vi "Actor Core.vi"(8 "error in":errorcluster, 11 "Assert in":refnum<class "Assert.lvclass">) -> (0 "error out":errorcluster, 3 "Actor out":refnum<class "Actor.lvclass">)   [LabVIEW 2019, in "Assert.lvlib" / "Assert.lvclass"]
doc: "(<B>Filename</B>: Actor Framework.lvlib:Actor.lvclass:Actor Core.vi)\n\nReceives messages to the actor, reacts to them, and initiates any error handling that may shut the actor down.\n\nDescendant classes may override this VI to append parallel tasks for the actor to complete while it handles messages. Overrides use the Call Parent Method node."
uses:
  Assert.lvclass
  C:/Program Files (x86)/National Instruments/LabVIEW 2019/vi.lib/ActorFramework/Actor/Actor.lvclass
  <vilib>/ActorFramework/Actor/Actor.lvclass
  Assert.lvclass/Assert.ctl
  <vilib>/ActorFramework/Actor/Actor.lvclass/Actor.ctl
  <vilib>/ActorFramework/Message Enqueuer/Message Enqueuer.lvclass/Message Enqueuer.ctl
  Assert Event.lvclass
  C:/Program Files (x86)/National Instruments/LabVIEW 2019/vi.lib/NI/Event Source Actor/Event Source/Event/Event.lvclass
  <vilib>/NI/Event Source Actor/Event Source/Event/Event.lvclass/Event.ctl
  <vilib>/NI/Event Source Actor/Event Source/Event Source Messages/Generate Event Msg/Generate Event Msg.lvclass/Generate Event Msg.ctl
  <vilib>/ActorFramework/Message Enqueuer/Init from Existing Queue.vi
  <vilib>/ActorFramework/Message Enqueuer/Enqueue.vi
  <vilib>/NI/Event Source Actor/Event Source/Event Source Messages/Generate Event Msg/Generate Event Msg.lvclass
  C:/Program Files (x86)/National Instruments/LabVIEW 2019/vi.lib/ActorFramework/Message/Message.lvclass
  Unit Test Engine Global.vi
  <vilib>/ActorFramework/Message Priority Queue/Priority Enqueue.vi
  <vilib>/NI/Event Source Actor/Event Source/Event Source/Event Source.lvclass
  <vilib>/ActorFramework/Message Enqueuer/Message Enqueuer.lvclass
  Assert.lvlib
  <vilib>/NI/Event Source Actor/Event Source/Event/Event.lvclass
panel:
  out "StartTime":u32
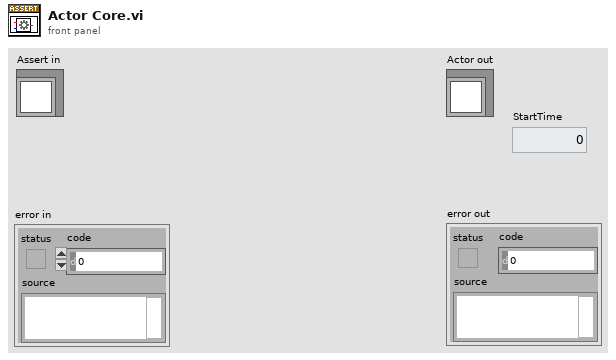
[diagram p1: front panel]
types:
  T1 = cluster{"Socket":i32, "Result":string, "Value":string, "Limit":cluster{"High":string, "Low":string}, "Type":string, "StepName":string, "Normal":string, "Unit":string}
  T2 = cluster{"Socket":i32, "StepName":string, "Sequence":string}
  T3 = enum32{"Invalid", "Standard", "Closed", "Hidden", "Minimized", "Maximized"}
  T4 = enum32{"invalid app kind", "Development System", "Run Time System", "Student Edition", "Embedded LabVIEW", "Evaluation", "Custom"}
  T5 = cluster{"Core":cluster{"Current VI Reference":refnum<vi>, "Close Panel on Exit?":bool}, "Your Boolean data":bool, "Your string data":string}
  T6 = cluster{"Current VI Reference":refnum<vi>, "Close Panel on Exit?":bool}
  T7 = cluster{"Socket":i32, "StepName":string, "Sequence":string}[]
  T8 = cluster{"Socket":i32, "Result":string, "Value":string, "Limit":cluster{"High":string, "Low":string}, "Type":string, "StepName":string, "Normal":string, "Unit":string}[]
  T9 = cluster{cluster{"Socket":i32, "Result":string, "Value":string, "Limit":cluster{"High":string, "Low":string}, "Type":string, "StepName":string, "Normal":string, "Unit":string}[], dbl}
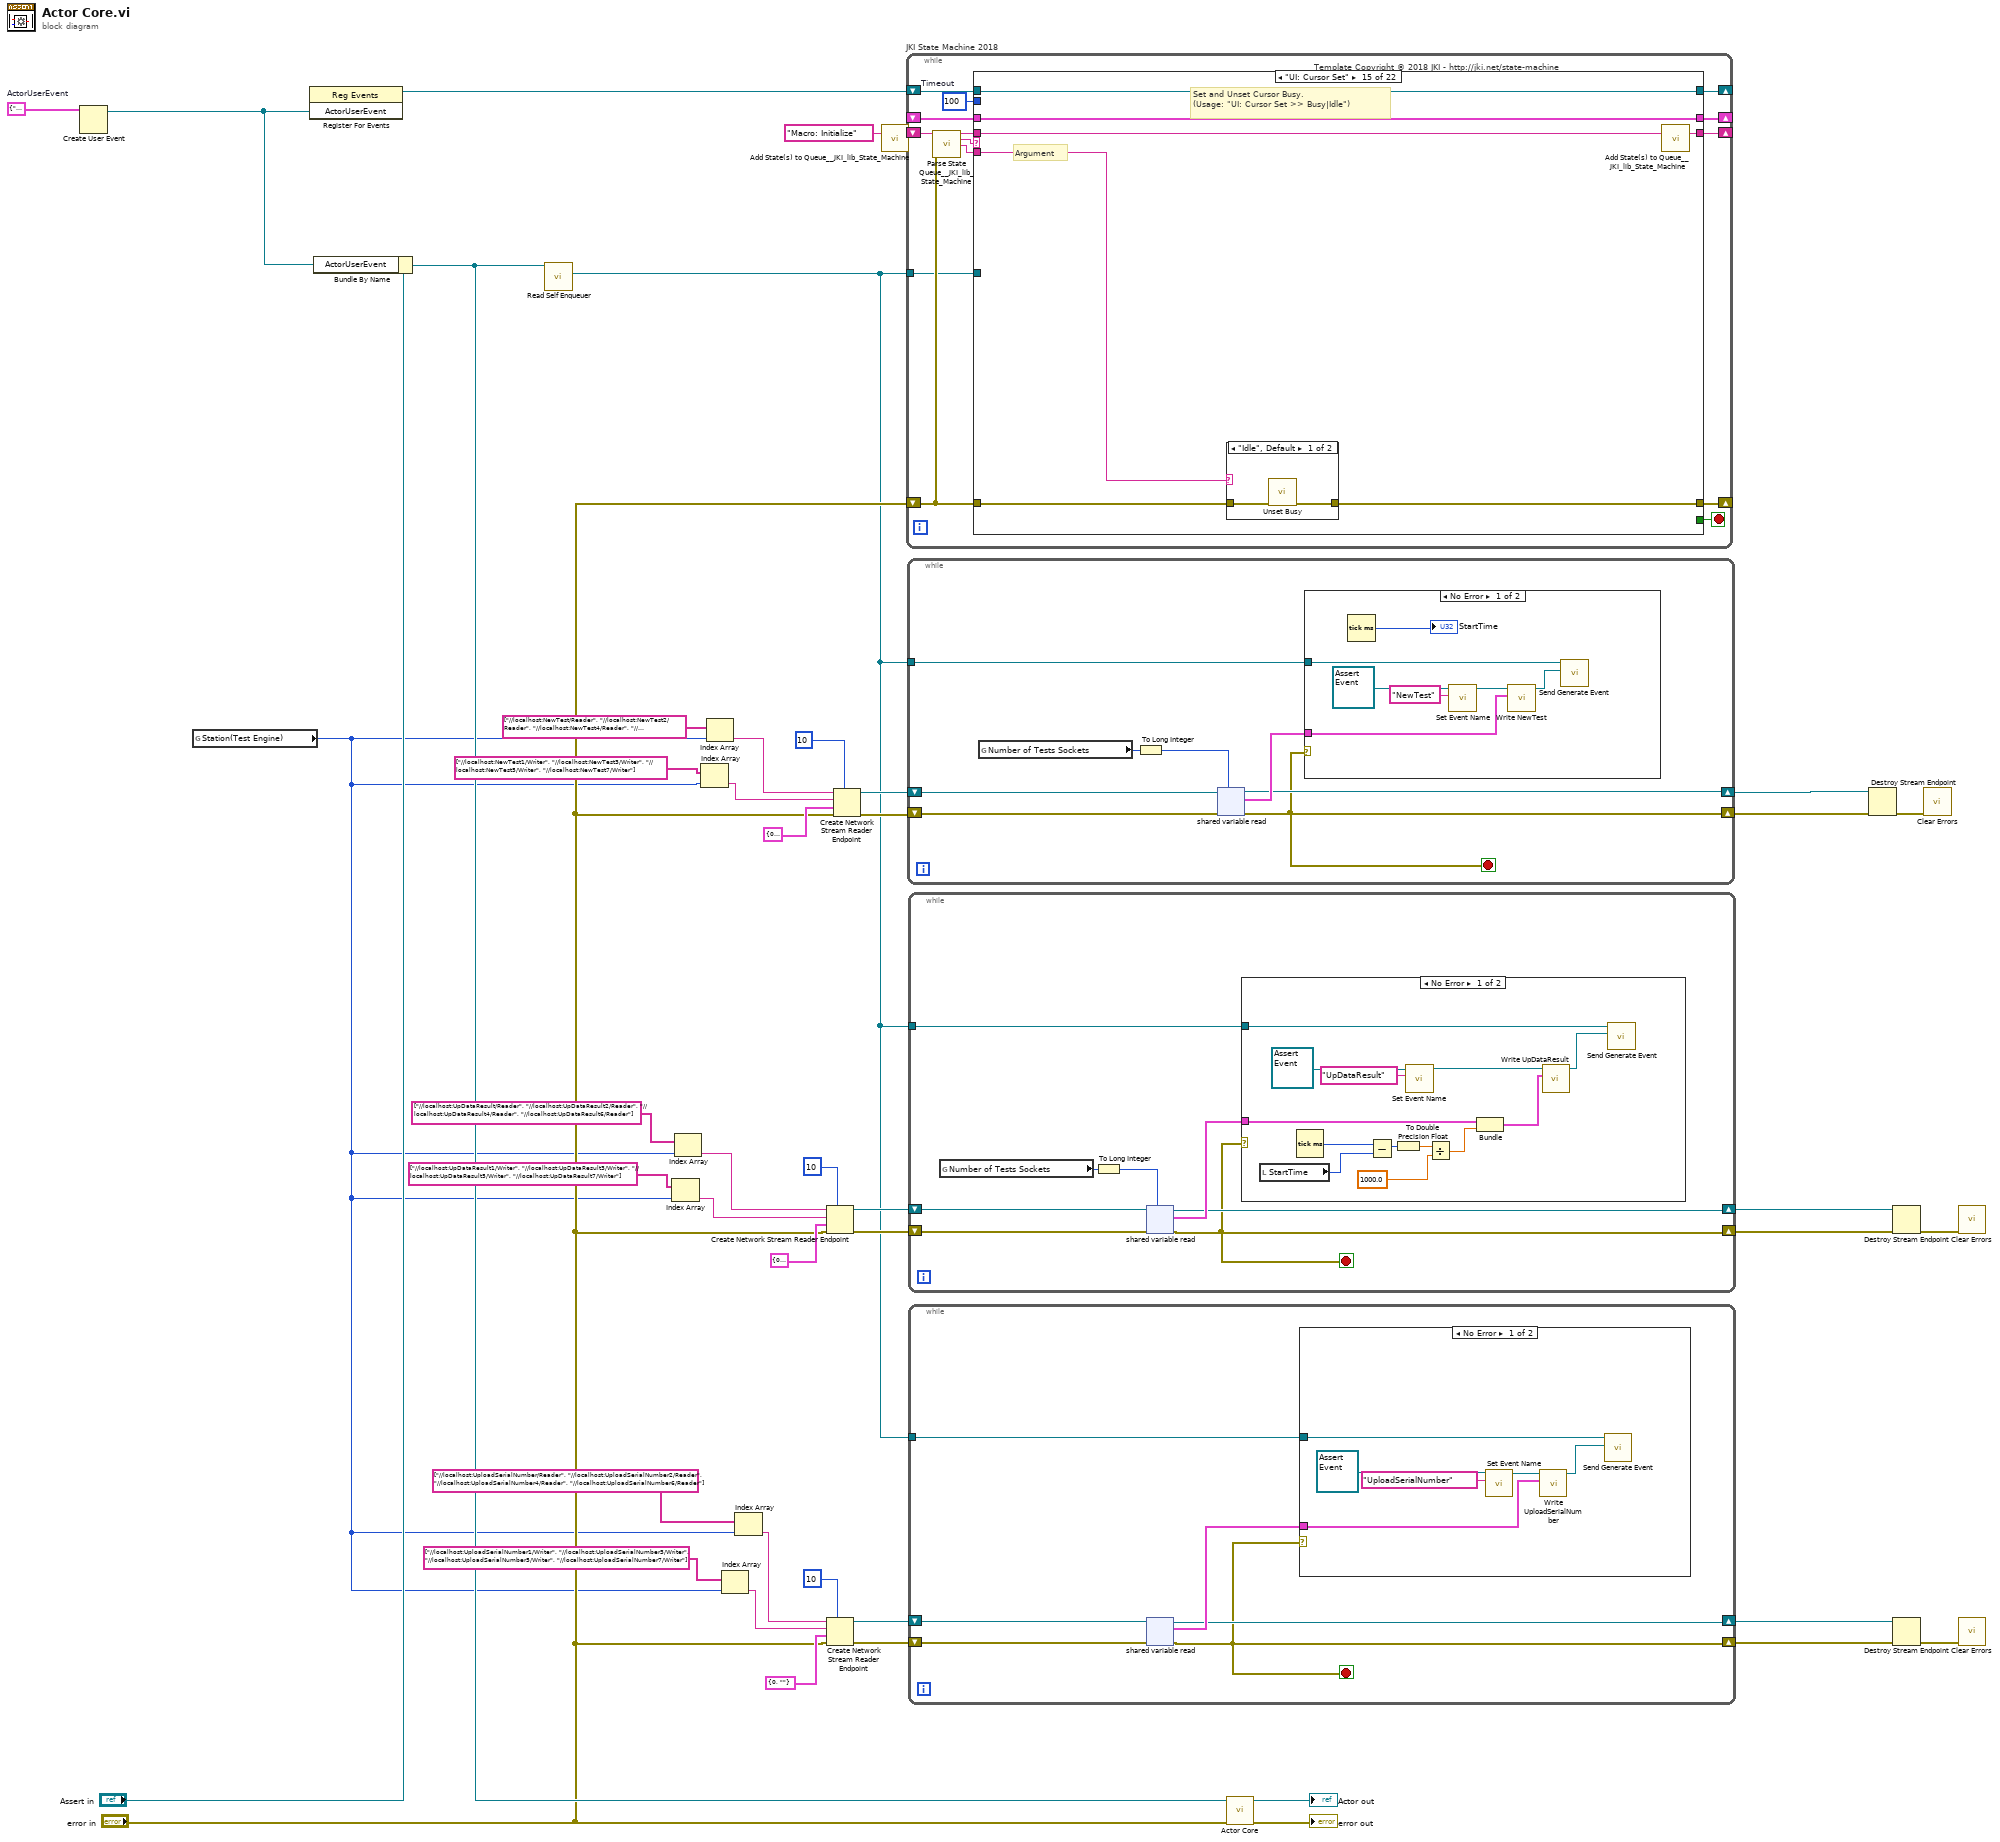
[diagram p0: block diagram]
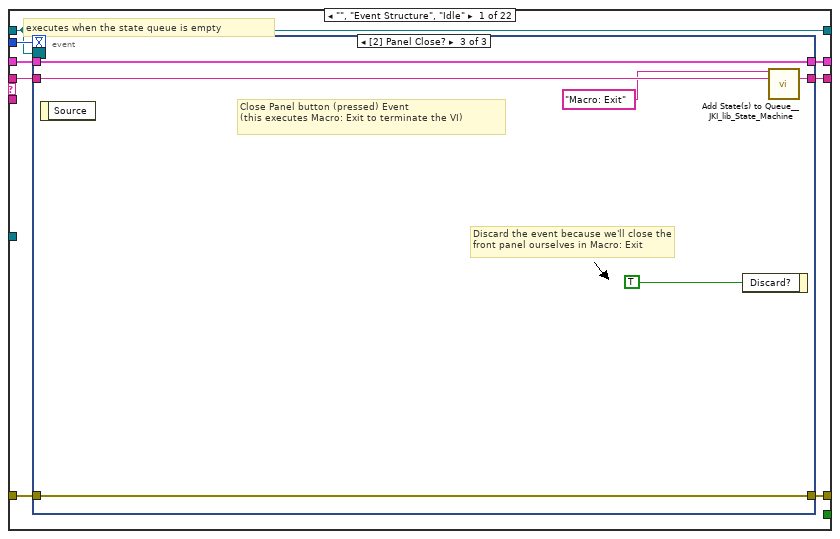
[diagram p5: hidden frame]
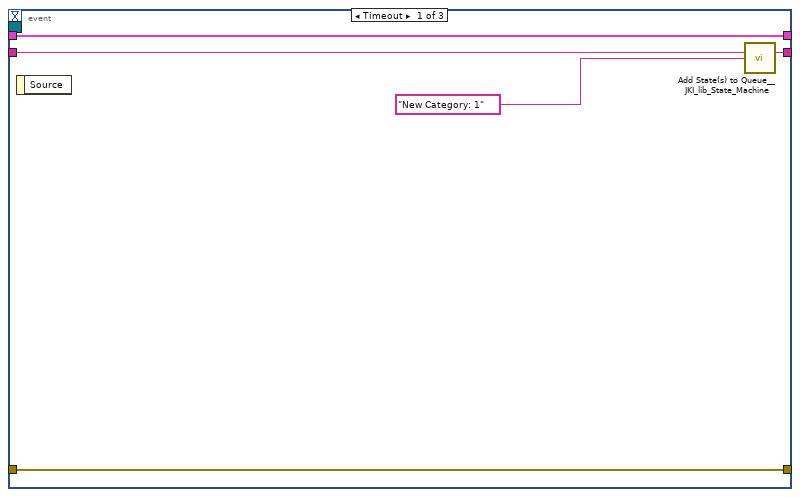
[diagram p6: hidden frame]
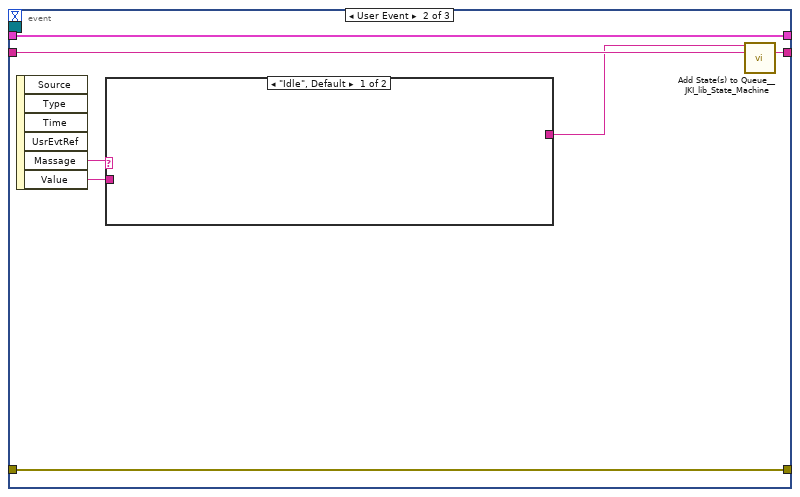
[diagram p7: hidden frame]
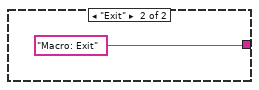
[diagram p8: hidden frame]
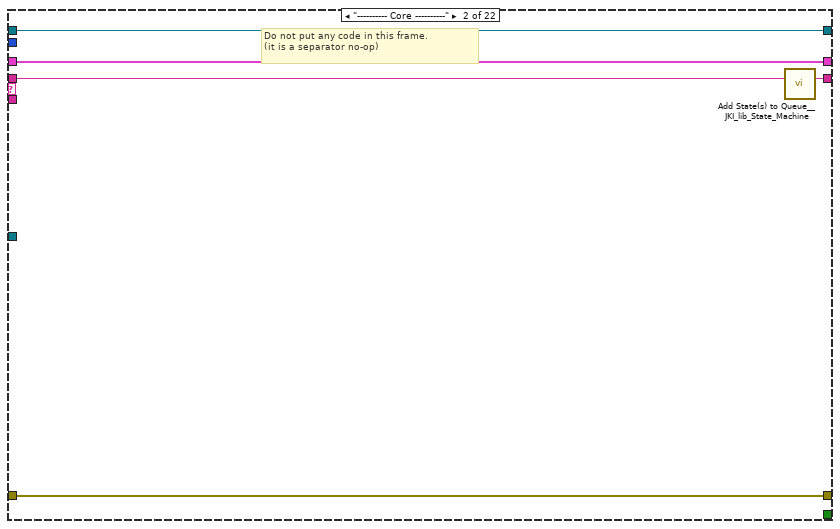
[diagram p9: hidden frame]
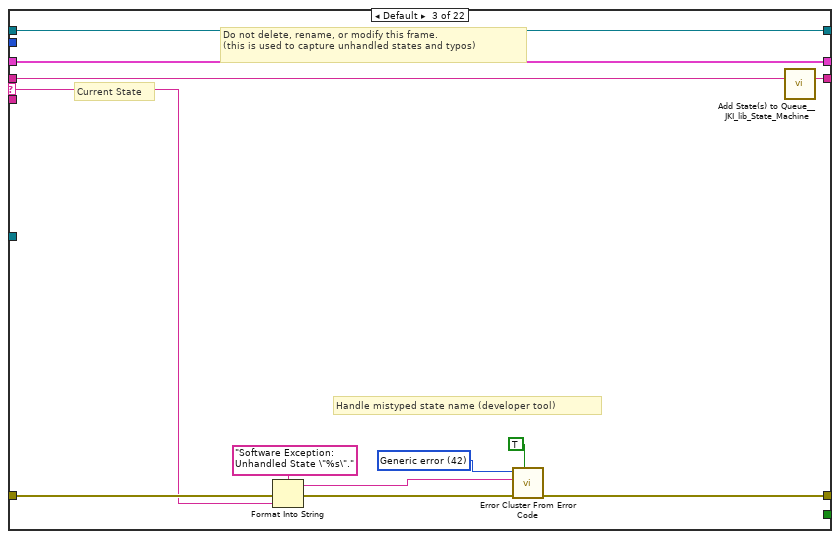
[diagram p10: hidden frame]
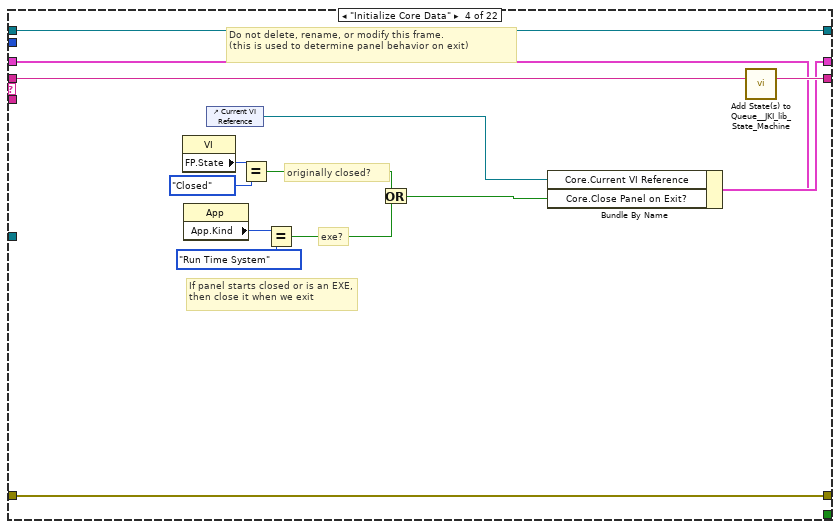
[diagram p11: hidden frame]
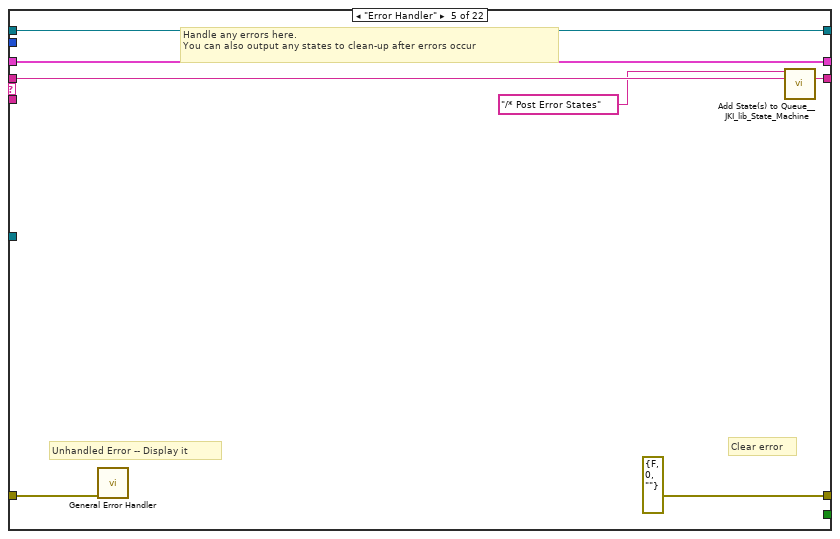
[diagram p12: hidden frame]
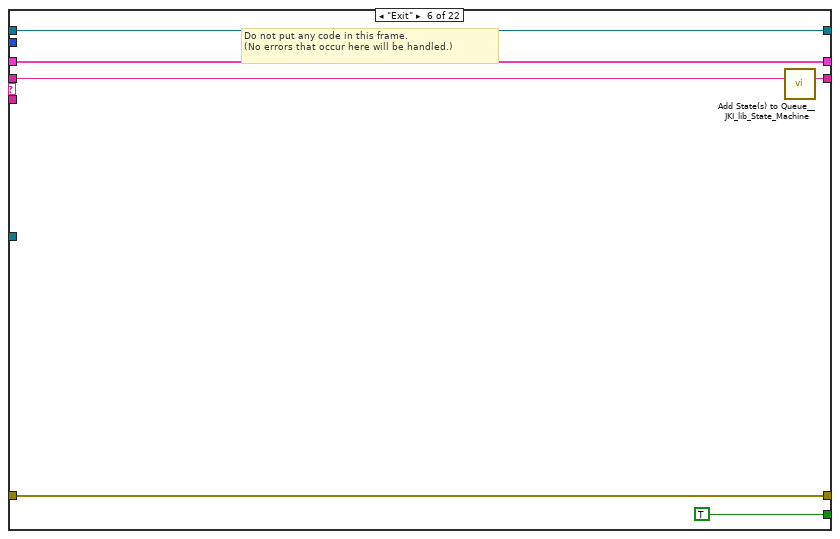
[diagram p13: hidden frame]
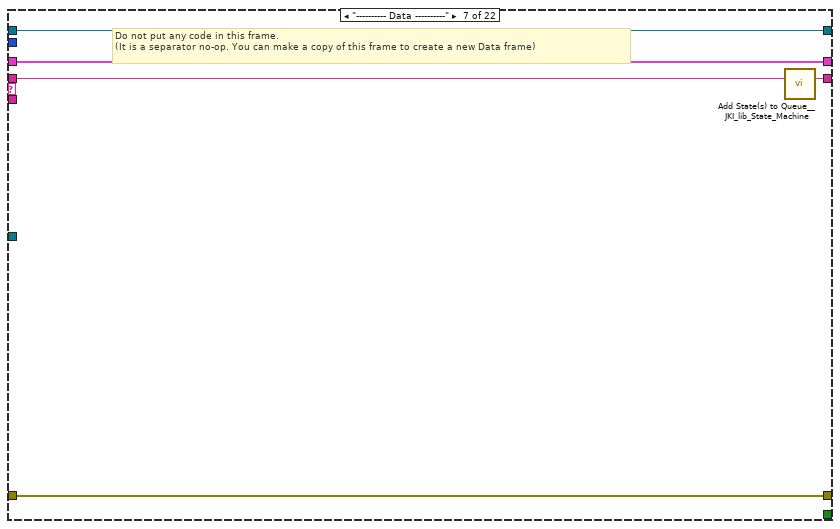
[diagram p14: hidden frame]
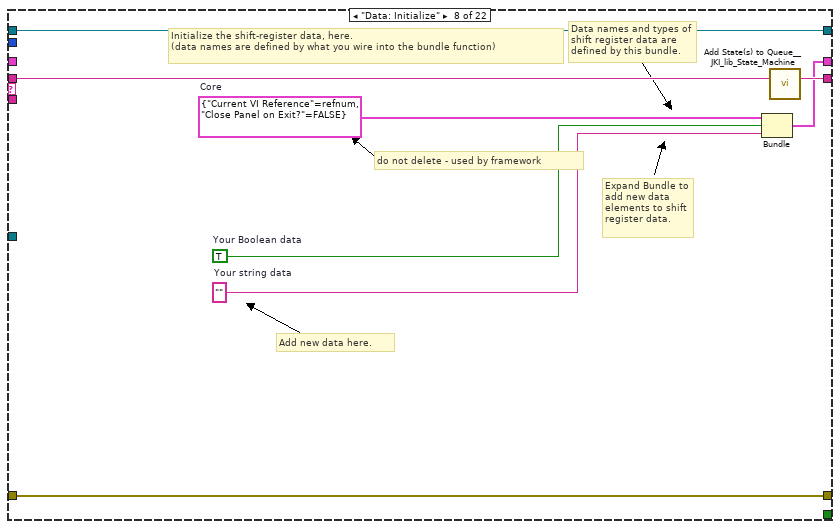
[diagram p15: hidden frame]
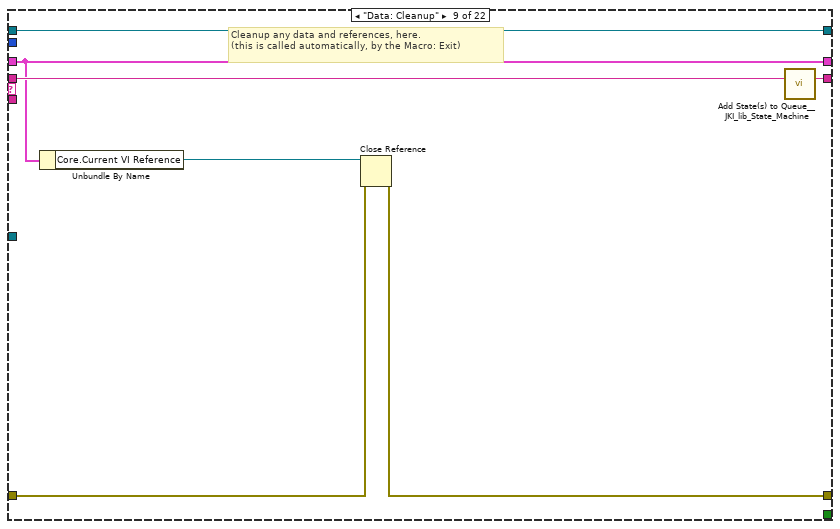
[diagram p16: hidden frame]
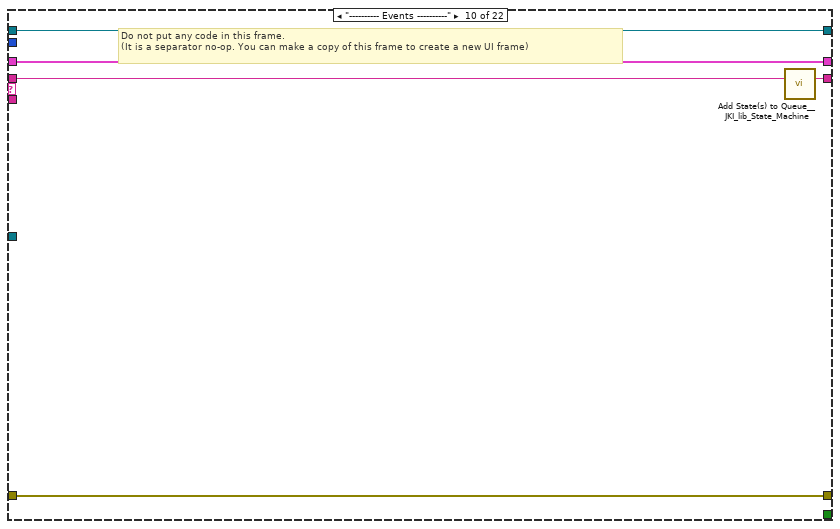
[diagram p17: hidden frame]
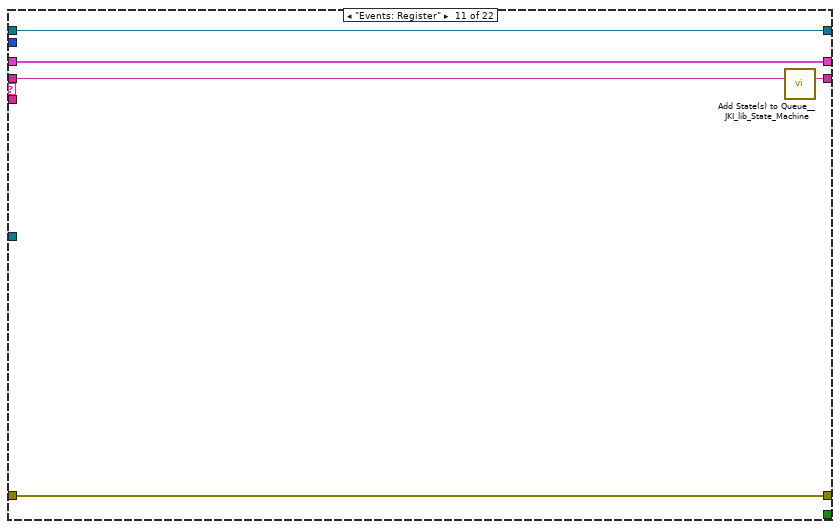
[diagram p18: hidden frame]
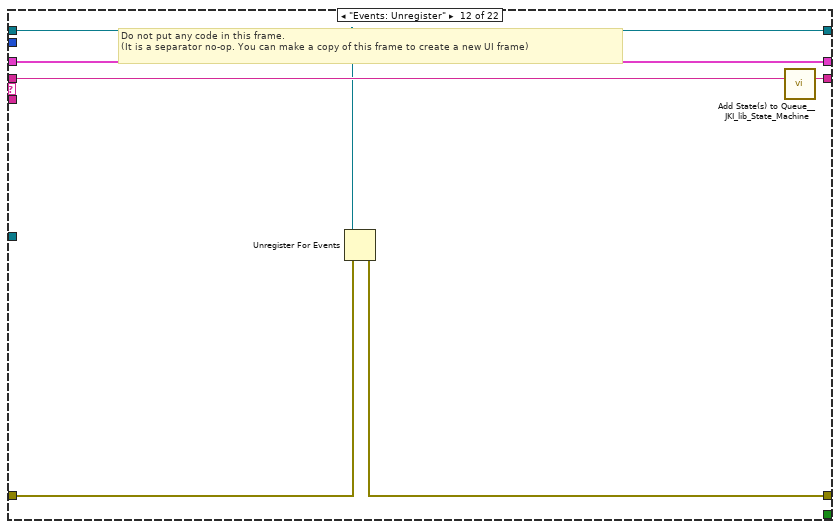
[diagram p19: hidden frame]
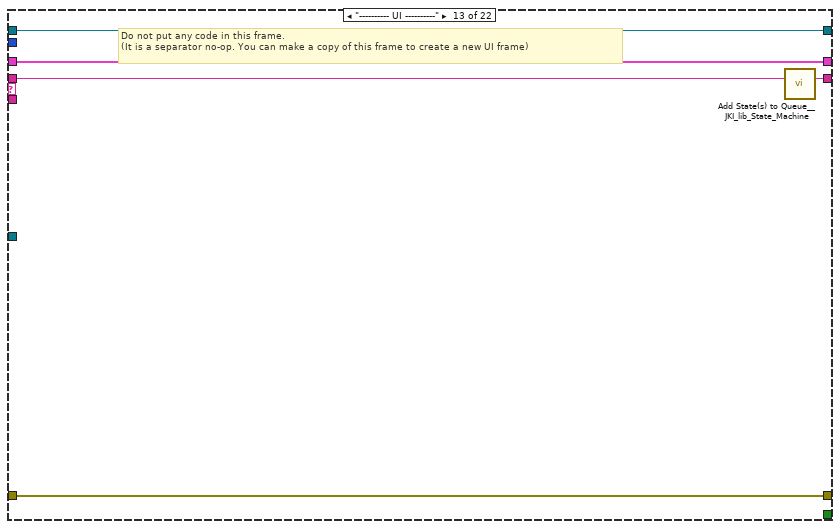
[diagram p20: hidden frame]
diagram:
  w41 = cluster{"Massage":string, "Value":string} {"Massage"="", "Value"=""}  # ActorUserEvent
  n1 = Create User Event(user event datatype=w41) -> (user event=w38:refnum<user-event>)  [unwired: 1 in, 1 out]
  n2 = global read "Unit Test Engine Global.vi" "Station(Test Engine)"() -> (w3:i32)
  n3 = register-events(w38) -> (reference out=w40:refnum<event-registration>)  [unwired: 2 in, 1 out]
  n4 = Bundle By Name(cluster="Assert in", "ActorUserEvent"=w38) -> (w16:refnum<class "Assert.lvclass">)
  n5 = call <vilib>:"Read Self Enqueuer.vi"("Actor"=w16) -> ("Self Enqueuer"=w1:refnum<class "Message Enqueuer.lvclass">)  [unwired: 10 in]
  n6 = Index Array(array=string[] ["//localhost:UpDataResult1/Writer", "//localhost:UpDataResult3/Writer", "//localhost:UpDataResult5/Writer", "//localhost:UpDataResult7/Writer"], index=w3) -> (element=w7:string)
  n7 = Index Array(array=string[] ["//localhost:UpDataResult/Reader", "//localhost:UpDataResult2/Reader", "//localhost:UpDataResult4/Reader", "//localhost:UpDataResult6/Reader"], index=w3) -> (element=w11:string)
  n8 = Index Array(array=string[] ["//localhost:NewTest1/Writer", "//localhost:NewTest3/Writer", "//localhost:NewTest5/Writer", "//localhost:NewTest7/Writer"], index=w3) -> (element=w2:string)
  n9 = Index Array(array=string[] ["//localhost:NewTest/Reader", "//localhost:NewTest2/Reader", "//localhost:NewTest4/Reader", "//localhost:NewTest6/Reader"], index=w3) -> (element=w13:string)
  n10 = Index Array(array=string[] ["//localhost:UploadSerialNumber1/Writer", "//localhost:UploadSerialNumber3/Writer", "//localhost:UploadSerialNumber5/Writer", "//localhost:UploadSerialNumber7/Writer"], index=w3) -> (element=w5:string)
  n11 = Index Array(array=string[] ["//localhost:UploadSerialNumber/Reader", "//localhost:UploadSerialNumber2/Reader", "//localhost:UploadSerialNumber4/Reader", "//localhost:UploadSerialNumber6/Reader"], index=w3) -> (element=w9:string)
  n12 = Create Network Stream Reader Endpoint(7:10 ("reader buffer size"), 8:"error in", 9:T1 {"Socket"=0, "Result"="", "Value"="", "Limit"={"High"="", "Low"=""}, "Type"="", "StepName"="", "Normal"="", "Unit"=""}, 10:w7, 11:w11) -> (0:w27:errorcluster, 3:w26:refnum<k21>)  [unwired: 2 in]
  n13 = Create Network Stream Reader Endpoint(7:10 ("reader buffer size"), 8:"error in", 9:cluster{"Socket":i32, "SerialNumber":string} {"Socket"=0, "SerialNumber"=""}, 10:w5, 11:w9) -> (0:w21:errorcluster, 3:w22:refnum<k21>)  [unwired: 2 in]
  n14 = Create Network Stream Reader Endpoint(7:10 ("reader buffer size"), 8:"error in", 9:T2 {"Socket"=0, "StepName"="", "Sequence"=""}, 10:w2, 11:w13) -> (0:w33:errorcluster, 3:w32:refnum<k21>)  [unwired: 2 in]
  n15 = call <vilib>:"Add State(s) to Queue__JKI_lib_State_Machine.vi"("State(s) in (\"\")"="Macro: Initialize") -> ("States Out"=w43:string)  [unwired: 14 in]
  n16 = while "JKI State Machine 2018" {
    shift-right: [w52] -> _
    shift-left: _ -> [w51]
    shift-right: [w55] -> _
    shift-left: "error in" -> [w49]
    shift-right: [w54] -> _
    shift-left: w43 -> [w56]
    shift-right: [w48] -> _
    shift-left: w40 -> [w47]
    tunnel: w1 -> [w46]
    stop <- w53 stop-if-true
    w50 = 100  # Timeout
    # "Template Copyright © 2018 JKI - http://jki.net/state-machine"
    n17 = call <vilib>:"Parse State Queue__JKI_lib_State_Machine.vi"("State Queue"=w56, "Error In (no error)"=w49) -> ("Remaining States"=w58:string, "Current State"=w59:string, "Arguments"=w57:string)  [unwired: 11 in]
    n18 = case shown="\"UI: Cursor Set\"" w59 {
      selector: w59 -> [_ _ w93 _ _ _ _ _ _ _ _ _ _ _ _ _ _ _ _ _ _ _]
      tunnel: w58 -> [w67 w91 w97 w117 w124 w130 w135 w143 w150 w155 w160 w166 w171 w176 w183 w195 w265 w271 w282 w287 w292 w297]
      tunnel: w57 -> [_ _ _ _ _ _ _ _ _ _ _ _ _ _ w178 w189 _ _ _ _ _ _]
      tunnel: w51 -> [w65 w88 w95 w110 w121 w128 w132 _ w145 w152 w158 w164 w168 w174 w181 w191 w262 w268 w279 w284 w290 w294]
      tunnel: [w64 w89 w99 w114 errorcluster {"status"=FALSE, "code"=0, "source"=""} ("error out") w127 w133 w140 w146 w153 w157 w161 w169 w173 w179 w192 w263 w269 w280 w285 w288 w295] -> w55
      tunnel: w49 -> [w63 w89 w98 w114 w120 w127 w133 w140 w147 w153 w157 w162 w169 w173 w180 w193 w263 w269 w280 w285 w288 w295]
      tunnel: [w66 w90 w96 w116 w123 w129 w134 w142 w149 w154 w159 w165 w170 w175 w182 w194 w264 w270 w281 w286 w291 w296] -> w54
      tunnel: [_ _ _ _ _ TRUE _ _ _ _ _ _ _ _ _ _ _ _ _ _ _ _] -> w53
      tunnel: [w62 w88 w95 w115 w121 w128 w132 w141 w145 w152 w158 w164 w168 w174 w181 w191 w262 w268 w279 w284 w290 w294] -> w52
      tunnel: w50 -> [w61 _ _ _ _ _ _ _ _ _ _ _ _ _ _ _ _ _ _ _ _ _]
      tunnel: [w60 w87 w92 w104 w118 w125 w131 w136 w144 w151 w156 w163 w167 w172 w177 w188 w261 w266 w272 w283 w289 w293] -> w48
      tunnel: w47 -> [w60 w87 w92 w104 w118 w125 w131 w136 w144 w151 w156 w163 w167 w172 w177 w188 w261 w266 w272 w283 w289 w293]
      tunnel: w46 -> [_ _ _ _ _ _ _ _ _ _ _ _ _ _ _ _ _ _ _ _ _ _]
      frame "", "Event Structure", "Idle" {
        # "executes when the state queue is empty"
        n19 = event shown="[2] Panel Close?" {
          selector: w60 -> [_ _ _]
          dyn-events: _ -> [_ _ _]
          timeout: w61 -> [_ _ _]
          tunnel: w67 -> [w72 w79 w86]
          tunnel: [w71 w78 w85] -> w66
          tunnel: w65 -> [w69 w76 w83]
          tunnel: [w70 w77 w84] -> w64
          tunnel: w63 -> [w70 w77 w84]
          tunnel: [w69 w76 w83] -> w62
          event Timeout {
            n20 = event-data() -> ()  [unwired: 1 in, 1 out]
            n21 = call <vilib>:"Add State(s) to Queue__JKI_lib_State_Machine.vi"("State(s) in (\"\")"=w72, "State(s) at Back (\"\")"="New Category: 1" ("State(s) at Back (\"\")")) -> ("States Out"=w71:string)  [unwired: 13 in]
          }
          event User Event {
            n22 = event-data() -> ("Massage"=w75:string, "Value"=w73:string)  [unwired: 1 in, 4 out]
            n23 = case shown="\"Idle\", Default" w75 {
              tunnel: [_ "Macro: Exit"] -> w74
              tunnel: w73 -> [_ _]
              frame "Idle", Default {
              }
              frame "Exit" {
              }
            }
            n24 = call <vilib>:"Add State(s) to Queue__JKI_lib_State_Machine.vi"("State(s) in Front (\"\")"=w74, "State(s) in (\"\")"=w79) -> ("States Out"=w78:string)  [unwired: 13 in]
          }
          event Panel Close? {
            # "Discard the event because we'll close the front panel ourselves in Macro: Exit"
            # "Close Panel button (pressed) Event\n(this executes Macro: Exit to terminate the VI)"
            n25 = event-data() -> ()  [unwired: 1 in, 1 out]
            n26 = event-data("Discard?"=TRUE) -> ()  [unwired: 1 in, 1 out]
            n27 = call <vilib>:"Add State(s) to Queue__JKI_lib_State_Machine.vi"("State(s) in Front (\"\")"="Macro: Exit", "State(s) in (\"\")"=w86) -> ("States Out"=w85:string)  [unwired: 13 in]
          }
        }
      }
      frame "---------- Core ----------" {
        # "Do not put any code in this frame.\n(it is a separator no-op)"
        n28 = call <vilib>:"Add State(s) to Queue__JKI_lib_State_Machine.vi"("State(s) in (\"\")"=w91) -> ("States Out"=w90:string)  [unwired: 14 in]
      }
      frame Default {
        w102 = 42 items=["No error", "Argument error", "Memory is full", "Out of zone", "End of file", "File already open", "Generic file I/O error", "File not found", "File permission error", "Disk is full", "Duplicate path", "Too many files open", "System feature not enabled", "Resource file not found", "Cannot add resource", "Resource not found", "Image not found", "Image memory error", "Pen does not exist", "Config type invalid", "Config token not found", "Config parse error", "Config memory error", "Bad external code format", "Bad external code offset", "External code not present", "Null window", "Destroy window error", "Null menu", "Print aborted", "Bad print record", "Print driver error", "Windows error during printing", "Memory error during printing", "Print dialog error", "Generic print error", "Invalid device refnum", "Device not found", "Device parameter error", "Device unit error", "Cannot open device", "Device call aborted", "Generic error", "Cancelled by user", "Object ID too low", "Object ID too high", "Object not in heap", "Unknown heap", "Unknown object (invalid DefProc)", "Unknown object (DefProc not in table)", "Message out of range", "Invalid (null) method", "Unknown message", "Manager call not supported", "Bad address", "Network operation in progress", "Network operation timed out", "Connection is busy", "Network attribute not supported", "Network error", "Address in use", "System out of memory", "Connection aborted", "Connection refused", "Not connected", "Already connected", "Connection closed", "Initialization error (interapplication manager)", "Bad occurrence", "Wait on unbound occurrence handler", "Occurrence queue overflow", "Datalog type conflict", "Unused", "Unrecognized type (interapplication manager)", "Memory corrupt", "Failed to make temporary DLL", "Old CIN version", "Drag socket not found", "Failed to load drop-object", "Failed to register OLE object", "Failed to release OLE object", "Format specifier type mismatch", "Unknown format specifier", "Too few format specifiers", "Too many format specifiers", "Scan failed", "Newer CIN version", "Error converting to variant", "Runtime menu error", "Password tampered", "Variant attribute not found", "Incompatible variant data type", "Event data is not available", "Event Store is not present", "Occurrence is not found", "Event Queue is not created", "Event info is not available", "Refnum passed is NULL", "Error retrieving Class GUID", "Error retrieving CoClass GUID", "Error retrieving TypeLib GUID.", "Bad built application magic bytes.", "Specific driver is different from the specific driver associated with the Logical Name.", "There is no session opened to the class driver.", "Max Error", "MAX - Error with config objects", "MAX - Error loading configuration", "MAX - Group not supported"]
        # "Current State"
        # "Do not delete, rename, or modify this frame.\n(this is used to capture unhandled states and typos)"
        # "Handle mistyped state name (developer tool)"
        n29 = Format Into String(format string="Software Exception: Unhandled State \"%s\"." ("message"), error in=w98, w93) -> (resulting string=w101:string, error out=w100:errorcluster)  [unwired: 1 in]
        n30 = call <vilib>:"Error Cluster From Error Code.vi"("show call chain? (False)"=TRUE, "error in (no error)"=w100, "error message (\"\")"=w101, "error code (0)"=w102) -> ("error out"=w99:errorcluster)  [unwired: 5 in]
        n31 = call <vilib>:"Add State(s) to Queue__JKI_lib_State_Machine.vi"("State(s) in (\"\")"=w97) -> ("States Out"=w96:string)  [unwired: 14 in]
      }
      frame "Initialize Core Data" {
        # "Do not delete, rename, or modify this frame.\n(this is used to determine panel behavior on exit)"
        # "originally closed?"
        # "exe?"
        # "If panel starts closed or is an EXE, then close it when we exit"
        n32 = property class="VI"() -> ("FP.State"=w107:T3)  [unwired: 2 in, 2 out]
        n33 = property class="App"() -> ("App.Kind"=w113:T4)  [unwired: 2 in, 2 out]
        n34 = control-ref of="Current VI Reference"() -> (w108:refnum<vi>)
        n35 = Equal?(x=w107, y=T3."Closed" ("Front Panel Window:State")) -> (x = y?=w105:bool)
        n36 = Equal?(x=w113, y=T4."Run Time System" ("Application:Kind")) -> (x = y?=w111:bool)
        n37 = Or(x=w105, y=w111) -> (x .or. y?=w109:bool)
        n38 = Bundle By Name(cluster=w110, "Core.Current VI Reference"=w108, "Core.Close Panel on Exit?"=w109) -> (w115:T5)
        n39 = call <vilib>:"Add State(s) to Queue__JKI_lib_State_Machine.vi"("State(s) in (\"\")"=w117) -> ("States Out"=w116:string)  [unwired: 14 in]
      }
      frame "Error Handler" {
        # "Unhandled Error -- Display it"
        # "Handle any errors here.\nYou can also output any states to clean-up after errors occur"
        # "Clear error"
        n40 = call <vilib>:"General Error Handler.vi"("error in (no error)"=w120) -> ()  [unwired: 10 in, 5 out]
        n41 = call <vilib>:"Add State(s) to Queue__JKI_lib_State_Machine.vi"("State(s) in Front (\"\")"="/* Post Error States", "State(s) in (\"\")"=w124) -> ("States Out"=w123:string)  [unwired: 13 in]
      }
      frame "Exit" {
        # "Do not put any code in this frame.\n(No errors that occur here will be handled.)"
        n42 = call <vilib>:"Add State(s) to Queue__JKI_lib_State_Machine.vi"("State(s) in (\"\")"=w130) -> ("States Out"=w129:string)  [unwired: 14 in]
      }
      frame "---------- Data ----------" {
        # "Do not put any code in this frame.\n(It is a separator no-op. You can make a copy of this frame to create a new Data frame)"
        n43 = call <vilib>:"Add State(s) to Queue__JKI_lib_State_Machine.vi"("State(s) in (\"\")"=w135) -> ("States Out"=w134:string)  [unwired: 14 in]
      }
      frame "Data: Initialize" {
        w137 = T6 {"Current VI Reference"=refnum, "Close Panel on Exit?"=FALSE}  # Core
        w139 = TRUE  # Your Boolean data
        w138 = ""  # Your string data
        # "do not delete - used by framework"
        # "Expand Bundle to add new data elements to shift register data."
        # "Add new data here."
        # "Data names and types of shift register data are defined by this bundle."
        # "Initialize the shift-register data, here.\n(data names are defined by what you wire into the bundle function)"
        n44 = Bundle("Core"=w137, "Your Boolean data"=w139, "Your string data"=w138) -> (w141:T5)  [unwired: 1 in]
        n45 = call <vilib>:"Add State(s) to Queue__JKI_lib_State_Machine.vi"("State(s) in (\"\")"=w143) -> ("States Out"=w142:string)  [unwired: 14 in]
      }
      frame "Data: Cleanup" {
        # "Cleanup any data and references, here.\n(this is called automatically, by the Macro: Exit)"
        n46 = Unbundle By Name(w145) -> ("Core.Current VI Reference"=w148:refnum<vi>)
        n47 = Close Reference(reference=w148, error in (no error)=w147) -> (error out=w146:errorcluster)
        n48 = call <vilib>:"Add State(s) to Queue__JKI_lib_State_Machine.vi"("State(s) in (\"\")"=w150) -> ("States Out"=w149:string)  [unwired: 14 in]
      }
      frame "---------- Events ----------" {
        # "Do not put any code in this frame.\n(It is a separator no-op. You can make a copy of this frame to create a new UI frame)"
        n49 = call <vilib>:"Add State(s) to Queue__JKI_lib_State_Machine.vi"("State(s) in (\"\")"=w155) -> ("States Out"=w154:string)  [unwired: 14 in]
      }
      frame "Events: Register" {
        n50 = call <vilib>:"Add State(s) to Queue__JKI_lib_State_Machine.vi"("State(s) in (\"\")"=w160) -> ("States Out"=w159:string)  [unwired: 14 in]
      }
      frame "Events: Unregister" {
        # "Do not put any code in this frame.\n(It is a separator no-op. You can make a copy of this frame to create a new UI frame)"
        n51 = Unregister For Events(event registration refnum=w163, error in=w162) -> (error out=w161:errorcluster)
        n52 = call <vilib>:"Add State(s) to Queue__JKI_lib_State_Machine.vi"("State(s) in (\"\")"=w166) -> ("States Out"=w165:string)  [unwired: 14 in]
      }
      frame "---------- UI ----------" {
        # "Do not put any code in this frame.\n(It is a separator no-op. You can make a copy of this frame to create a new UI frame)"
        n53 = call <vilib>:"Add State(s) to Queue__JKI_lib_State_Machine.vi"("State(s) in (\"\")"=w171) -> ("States Out"=w170:string)  [unwired: 14 in]
      }
      frame "UI: Initialize" {
        # "Initialize the User Interface, here.\n(this is called automatically, by the Macro: Init)"
        n54 = call <vilib>:"Add State(s) to Queue__JKI_lib_State_Machine.vi"("State(s) in (\"\")"=w176) -> ("States Out"=w175:string)  [unwired: 14 in]
      }
      frame "UI: Cursor Set" {
        # "Argument"
        # "Set and Unset Cursor Busy.\n(Usage: \"UI: Cursor Set >> Busy|Idle\")"
        n55 = case shown="\"Idle\", Default" w178 {
          tunnel: w180 -> [w185 w187]
          tunnel: [w184 w186] -> w179
          frame "Idle", Default {
            n56 = call <vilib>:"Unset Busy.vi"("error in (no error)"=w185) -> ("error out"=w184:errorcluster)  [unwired: 10 in]
          }
          frame "Busy" {
            n57 = call <vilib>:"Set Busy.vi"("error in (no error)"=w187) -> ("error out"=w186:errorcluster)  [unwired: 9 in, 1 out]
          }
        }
        n58 = call <vilib>:"Add State(s) to Queue__JKI_lib_State_Machine.vi"("State(s) in (\"\")"=w183) -> ("States Out"=w182:string)  [unwired: 14 in]
      }
      frame "UI: Front Panel State" {
        # "Argument"
        # "Set Front Panel Open or Closed\n(Usage: \"UI: Front Panel State >> Open|Close\")"
        n59 = Unbundle By Name(w191) -> ("Core.Current VI Reference"=w190:refnum<vi>)
        n60 = case shown="\"Minimize\", \"Minimized\"" w189 {
          tunnel: w193 -> [w201 w216 w227 w240 w253]
          tunnel: [w203 w217 w229 w242 w255] -> w192
          tunnel: w190 -> [w202 w214 w228 w241 w254]
          frame "Open", "Standard", Default {
            w196 = T3."Standard" ("State")
            n61 = property class="VI"(reference=w202, error in=w201) -> (reference out=w199:refnum<vi>, error out=w200:errorcluster, "FP.State"=w198:T3)
            n62 = Not Equal?(x=w198, y=w196) -> (x != y?=w197:bool)
            n63 = case shown="True" w197 {
              tunnel: [w207 w209] -> w203
              tunnel: w200 -> [w206 w209]
              tunnel: w199 -> [w205 _]
              tunnel: w196 -> [w204 _]
              frame True {
                n64 = invoke class="VI" method="FP.Open"(reference=w205, error in=w206, "Activate"=TRUE, "State"=w204) -> (error out=w207:errorcluster)  [unwired: 1 in, 4 out]
              }
              frame False {
              }
            }
          }
          frame "Close", "Closed" {
            n65 = property class="VI"(reference=w214, error in=w216) -> (reference out=w213:refnum<vi>, error out=w215:errorcluster, "FP.State"=w211:T3)
            n66 = Not Equal?(x=w211, y=T3."Closed" ("Front Panel Window:State")) -> (x != y?=w210:bool)
            n67 = case shown="True" w210 {
              tunnel: [w218 w221] -> w217
              tunnel: w215 -> [w218 w220]
              tunnel: w213 -> [_ w219]
              frame False {
              }
              frame True {
                n68 = invoke class="VI" method="FP.Close"(reference=w219, error in=w220) -> (error out=w221:errorcluster)  [unwired: 1 in, 2 out]
              }
            }
          }
          frame "Hidden", "Hide" {
            w222 = T3."Hidden" ("State")
            n69 = property class="VI"(reference=w228, error in=w227) -> (reference out=w225:refnum<vi>, error out=w226:errorcluster, "FP.State"=w224:T3)
            n70 = Not Equal?(x=w224, y=w222) -> (x != y?=w223:bool)
            n71 = case shown="True" w223 {
              tunnel: [w233 w234] -> w229
              tunnel: w226 -> [w232 w234]
              tunnel: w225 -> [w231 _]
              tunnel: w222 -> [w230 _]
              frame True {
                n72 = invoke class="VI" method="FP.Open"(reference=w231, error in=w232, "State"=w230) -> (error out=w233:errorcluster)  [unwired: 2 in, 4 out]
              }
              frame False {
              }
            }
          }
          frame "Minimize", "Minimized" {
            w235 = T3."Minimized" ("State")
            n73 = property class="VI"(reference=w241, error in=w240) -> (reference out=w238:refnum<vi>, error out=w239:errorcluster, "FP.State"=w237:T3)
            n74 = Not Equal?(x=w237, y=w235) -> (x != y?=w236:bool)
            n75 = case shown="True" w236 {
              tunnel: [w246 w247] -> w242
              tunnel: w239 -> [w245 w247]
              tunnel: w238 -> [w244 _]
              tunnel: w235 -> [w243 _]
              frame True {
                n76 = invoke class="VI" method="FP.Open"(reference=w244, error in=w245, "State"=w243) -> (error out=w246:errorcluster)  [unwired: 2 in, 4 out]
              }
              frame False {
              }
            }
          }
          frame "Maximize", "Maximized" {
            w248 = T3."Maximized" ("State")
            n77 = property class="VI"(reference=w254, error in=w253) -> (reference out=w251:refnum<vi>, error out=w252:errorcluster, "FP.State"=w250:T3)
            n78 = Not Equal?(x=w250, y=w248) -> (x != y?=w249:bool)
            n79 = case shown="True" w249 {
              tunnel: [w259 w260] -> w255
              tunnel: w252 -> [w258 w260]
              tunnel: w251 -> [w257 _]
              tunnel: w248 -> [w256 _]
              frame True {
                n80 = invoke class="VI" method="FP.Open"(reference=w257, error in=w258, "State"=w256) -> (error out=w259:errorcluster)  [unwired: 2 in, 4 out]
              }
              frame False {
              }
            }
          }
        }
        n81 = call <vilib>:"Add State(s) to Queue__JKI_lib_State_Machine.vi"("State(s) in (\"\")"=w195) -> ("States Out"=w194:string)  [unwired: 14 in]
      }
      frame "---------- Macro ----------" {
        # "Do not put any code in this frame.\n(It is a separator no-op. You can make a copy of this frame to create a new Macro frame)"
        n82 = call <vilib>:"Add State(s) to Queue__JKI_lib_State_Machine.vi"("State(s) in (\"\")"=w265) -> ("States Out"=w264:string)  [unwired: 14 in]
      }
      frame "Macro: Initialize" {
        # "Initialization Macro\n(This is called once, when the VI starts)"
        n83 = call <vilib>:"Add State(s) to Queue__JKI_lib_State_Machine.vi"("State(s) in Front (\"\")"="Data: Initialize\nInitialize Core Data\nEvents: Register\nUI: Initialize\nUI: Front Panel State >> Close", "State(s) in (\"\")"=w271) -> ("States Out"=w270:string)  [unwired: 13 in]
      }
      frame "Macro: Exit" {
        # "Exit Macro\n(This is called once, when the VI exits)"
        n84 = Unbundle By Name(w279) -> ("Core.Close Panel on Exit?"=w278:bool)
        n85 = Select(t="UI: Front Panel State >> Close", s=w278, f="") -> (s? t:f=w275:string)
        n86 = call <vilib>:"Add State(s) to Queue__JKI_lib_State_Machine.vi"("State(s) in (\"\")"=w275, "State(s) at Back (\"\")"="Data: Cleanup\nEvents: Unregister\nExit") -> ("States Out"=w273:string)  [unwired: 13 in]
        n87 = call <vilib>:"Add State(s) to Queue__JKI_lib_State_Machine.vi"("State(s) in Front (\"\")"=w273, "State(s) in (\"\")"=w282) -> ("States Out"=w281:string)  [unwired: 13 in]
      }
      frame "---------- New Category ----------" {
        # "Template Separator\n(You can make a copy of, or modify, this frame)"
        n88 = call <vilib>:"Add State(s) to Queue__JKI_lib_State_Machine.vi"("State(s) in (\"\")"=w287) -> ("States Out"=w286:string)  [unwired: 14 in]
      }
      frame "New Category: 1" {
        n89 = call <vilib>:"Add State(s) to Queue__JKI_lib_State_Machine.vi"("State(s) in (\"\")"=w292) -> ("States Out"=w291:string)  [unwired: 14 in]
      }
      frame "New Category: 2" {
        # "Your code here.\n(You can make a copy of, or modify, this frame)"
        n90 = call <vilib>:"Add State(s) to Queue__JKI_lib_State_Machine.vi"("State(s) in (\"\")"=w297) -> ("States Out"=w296:string)  [unwired: 14 in]
      }
    }
  }
  n91 = while {
    shift-right: [w299] -> w36
    shift-left: w33 -> [w300]
    shift-right: [w302] -> w37
    shift-left: w32 -> [w301]
    tunnel: w1 -> [w298]
    stop <- w299 stop-if-true
    n92 = global read "Unit Test Engine Global.vi" "Number of Tests Sockets"() -> (w304:u8)
    n93 = To Long Integer(number=w304) -> (32bit integer=w303:i32)
    n94 = shared-variable-read(w301, w300, w303) -> (w302:refnum<k21>, w299:errorcluster, w305:T7)  [unwired: 1 in, 1 out]
    n95 = case shown="No Error" w299 {
      tunnel: w305 -> [w307 _]
      tunnel: w298 -> [w311 _]
      frame No Error {
        n96 = Tick Count (ms)() -> (millisecond timer value=→"StartTime":u32)
        n97 = call <vilib>:"Set Event Name.vi"("Name (Generic)"="NewTest", "Event In"=refnum<class "Assert Event.lvclass"> refnum ("Assert.lvlib:Assert Event.lvclass")) -> ("Event Out"=w308:refnum<class "Assert Event.lvclass">)  [unwired: 9 in]
        n98 = call-dynamic "Write NewTest.vi"("NewTest"=w307, "Assert Event in"=w308) -> ("Assert Event out"=w306:refnum<class "Assert Event.lvclass">)  [unwired: 8 in, 1 out]
        n99 = call <vilib>:"Send Generate Event.vi"("Event"=w306, "Event Source Address"=w311) -> ()  [unwired: 8 in, 2 out]
      }
      frame Error {
      }
    }
  }
  n100 = while {
    shift-right: [w314] -> w31
    shift-left: w27 -> [w315]
    shift-right: [w317] -> w30
    shift-left: w26 -> [w316]
    tunnel: w1 -> [w313]
    stop <- w314 stop-if-true
    n101 = global read "Unit Test Engine Global.vi" "Number of Tests Sockets"() -> (w319:u8)
    n102 = To Long Integer(number=w319) -> (32bit integer=w318:i32)
    n103 = shared-variable-read(w316, w315, w318) -> (w317:refnum<k21>, w314:errorcluster, w320:T8)  [unwired: 1 in, 1 out]
    n104 = case shown="No Error" w314 {
      tunnel: w313 -> [w326 _]
      tunnel: w320 -> [w325 _]
      frame No Error {
        n105 = local read "StartTime"() -> (w330:u32)
        n106 = Tick Count (ms)() -> (millisecond timer value=w331:u32)
        n107 = Subtract(x=w331, y=w330) -> (x-y=w333:u32)
        n108 = To Double Precision Float(number=w333) -> (double precision float=w332:dbl)
        n109 = call <vilib>:"Set Event Name.vi"("Name (Generic)"="UpDataResult", "Event In"=refnum<class "Assert Event.lvclass"> refnum ("Assert.lvlib:Assert Event.lvclass")) -> ("Event Out"=w323:refnum<class "Assert Event.lvclass">)  [unwired: 9 in]
        n110 = Divide(x=w332, y=1000.0) -> (x/y=w324:dbl)
        n111 = Bundle(w325, w324) -> (w322:T9)  [unwired: 1 in]
        n112 = call-dynamic "Write UpDataResult.vi"("UpDataResult"=w322, "Assert Event in"=w323) -> ("Assert Event out"=w321:refnum<class "Assert Event.lvclass">)  [unwired: 8 in, 1 out]
        n113 = call <vilib>:"Send Generate Event.vi"("Event"=w321, "Event Source Address"=w326) -> ()  [unwired: 8 in, 2 out]
      }
      frame Error {
      }
    }
  }
  n114 = while {
    tunnel: w1 -> [w339]
    shift-right: [w334] -> w17
    shift-left: w21 -> [w335]
    shift-right: [w337] -> w18
    shift-left: w22 -> [w336]
    stop <- w334 stop-if-true
    n115 = shared-variable-read(w336, w335) -> (w337:refnum<k21>, w334:errorcluster, w338:cluster{"Socket":i32, "SerialNumber":string})  [unwired: 1 in, 1 out]
    n116 = case shown="No Error" w334 {
      tunnel: w339 -> [w343 _]
      tunnel: w338 -> [w340 _]
      frame No Error {
        n117 = call <vilib>:"Set Event Name.vi"("Name (Generic)"="UploadSerialNumber", "Event In"=refnum<class "Assert Event.lvclass"> refnum ("Assert.lvlib:Assert Event.lvclass")) -> ("Event Out"=w342:refnum<class "Assert Event.lvclass">)  [unwired: 9 in]
        n118 = call-dynamic "Write UploadSerialNumber.vi"("UploadSerialNumber"=w340, "Assert Event in"=w342) -> ("Assert Event out"=w341:refnum<class "Assert Event.lvclass">)  [unwired: 8 in, 1 out]
        n119 = call <vilib>:"Send Generate Event.vi"("Event"=w341, "Event Source Address"=w343) -> ()  [unwired: 8 in, 2 out]
      }
      frame Error {
      }
    }
  }
  n120 = call-parent "Actor Core.vi"("error in"="error in", "Actor in"=w16) -> ("error out"=→"error out":errorcluster, "Actor out"=→"Actor out":refnum<class "Actor.lvclass">)  [unwired: 8 in]
  n121 = Destroy Stream Endpoint(8:w36, 11:w37) -> (0:w25:errorcluster)
  n122 = Destroy Stream Endpoint(8:w31, 11:w30) -> (0:w24:errorcluster)
  n123 = Destroy Stream Endpoint(8:w17, 11:w18) -> (0:w23:errorcluster)
  n124 = call <vilib>:"Clear Errors.vi"("error in (no error)"=w25) -> ()  [unwired: 5 in, 2 out]
  n125 = call <vilib>:"Clear Errors.vi"("error in (no error)"=w24) -> ()  [unwired: 5 in, 2 out]
  n126 = call <vilib>:"Clear Errors.vi"("error in (no error)"=w23) -> ()  [unwired: 5 in, 2 out]
